vi "QI_CloseCam.vi"(3 "error in (no error)":errorcluster, 4 "Camera Handle":u32, 5 "path to dll":path) -> (0 "error out":errorcluster, 1 "CloseCam err":i32, 2 "Camera Handle":u32)   [LabVIEW 2014]
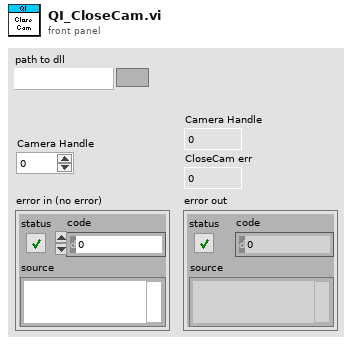
[diagram p1: front panel]
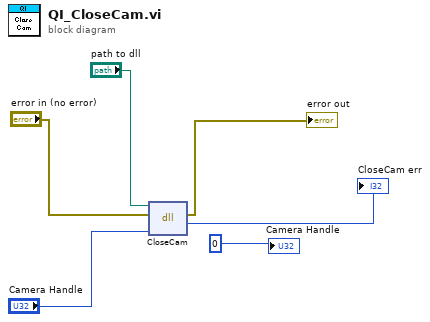
[diagram p0: block diagram]
diagram:
  n1 = dll-call lib="C:/Users/appli/Documents/Aline/octo-labview/QImaging/Release/QImaging.dll" fn="CloseCam"(path in="path to dll", error in="error in (no error)", "handle"="Camera Handle") -> (error out=→"error out":errorcluster, "return type"=→"CloseCam err":i32)  [unwired: 2 in, 1 out]
  "Camera Handle" <- u32 0
